vi "onCreate.vi"(8 "error in (no error)":errorcluster, 11 "RemoteControl.STM":refnum<class "RemoteControl.STM.lvclass">) -> (0 "error out":errorcluster, 3 "RemoteControl.STM out":refnum<class "RemoteControl.STM.lvclass">)   [LabVIEW 2019, in "RemoteControl.STM.lvclass"]
doc: "JKI State Machine Objects (SMO) 1.3.0.56\nJKI - JKI\nCopyright (c) 2017, JKI"
uses:
  RemoteControl.STM.lvclass
  RemoteControl/RemoteControl.lvclass
panel:
  # "For instructions on how to use the JKI State Machine Objects, examples and video tutorials, visit:\nhttp://jki.net/state-machine-objects/\n\nJKI State Machine Objects™\nhttp://jki.net/state-machine-objects/\nCopyright (C) 2005-2015, JKI <info@jki.net>\nALL RIGHTS RESERVED"
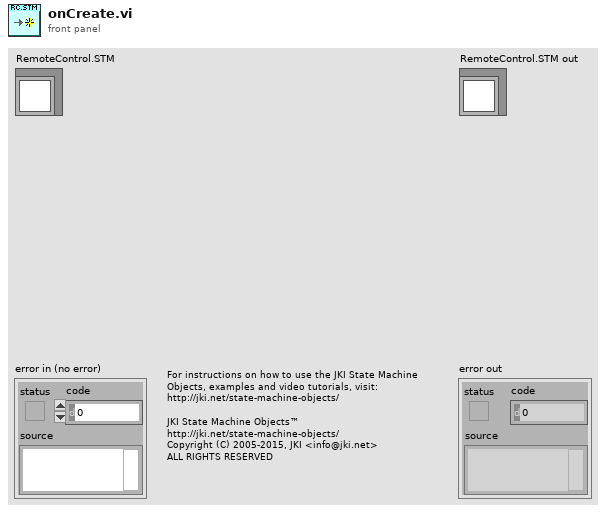
[diagram p1: front panel]
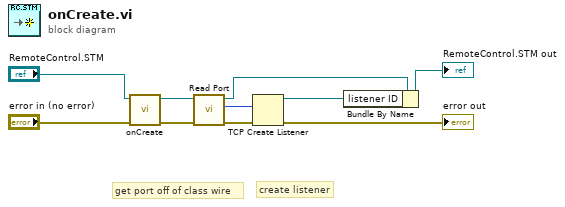
[diagram p0: block diagram]
diagram:
  # "get port off of class wire"
  # "create listener"
  n1 = call-parent "onCreate.vi"("error in (no error)"="error in (no error)", "SMO"="RemoteControl.STM") -> ("error out"=w5:errorcluster, "SMO out"=w6:refnum<class "RemoteControl.STM.lvclass">)  [unwired: 8 in]
  n2 = call-dynamic "Read Port.vi"("error in (no error)"=w5, "RemoteControl in"=w6) -> ("error out"=w8:errorcluster, "Port"=w7:u16, "RemoteControl out"=w4:refnum<class "RemoteControl.STM.lvclass">)  [unwired: 7 in]
  n3 = TCP Create Listener(8:w8, 10:w7) -> (0:→"error out":errorcluster, 3:w3:refnum<k5>)  [unwired: 3 in, 1 out]
  n4 = Bundle By Name(cluster=w4, "listener ID"=w3) -> (→"RemoteControl.STM out":refnum<class "RemoteControl.STM.lvclass">)
